vi "Periodic Tasks.vi"(8 "error in":errorcluster) -> ()   [LabVIEW 2019]
doc: "This VI runs in parallel to other tasks. It can contain as many user-defined periodic loops as you need. These can carry out PID or other sorts of timed response."
uses:
  <vilib>/Rock Robotics/WPI/Utilities/WPI_GetSetVariantRefNum.vi
  Robot Global Data.vi
  <vilib>/Rock Robotics/Network Tables/NT Read Boolean.vi
  <vilib>/Rock Robotics/WPI/RobotDrive/WPI_RobotDriveArcadeDrive_Standard(NoSaturation).vi
  <vilib>/Rock Robotics/Network Tables/NT Read Number.vi
  <vilib>/Rock Robotics/Network Tables/NT Write Numeric Array.vi
panel:
  in  "Target Y":dbl=1.0
  in  "Proportional Gain (X and Y)":dbl=0.25
  in  "Target X":dbl=1.0
  out "output":T1
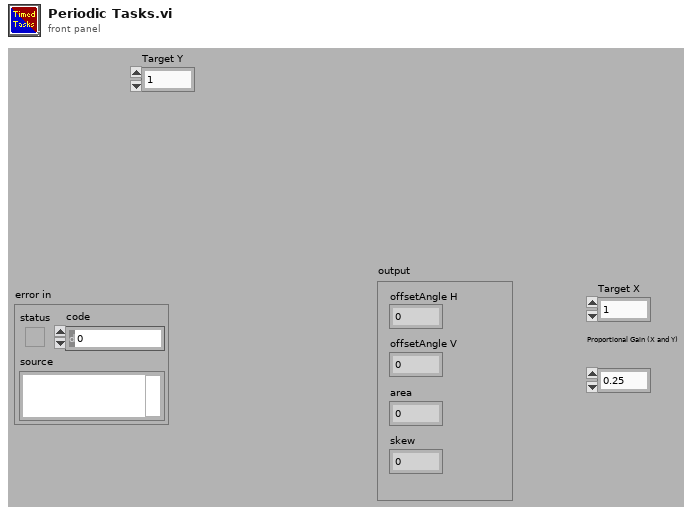
[diagram p1: front panel]
types:
  T1 = cluster{"offsetAngle H":dbl, "offsetAngle V":dbl, "area":dbl, "skew":dbl}
  T2 = typedef "WPI_JoystickDevRef.ctl" = cluster{"Device":T3}
  T3 = typedef "WPI_JoystickDeviceEnum.ctl" = enum16{"USB 0", "USB 1", "USB 2", "USB 3", "USB 4", "USB 5"}
  T4 = typedef "WPI_RobotDriveDevRef.ctl" = cluster{"DevStatus":errorcluster, "Motors[]":T5[], "Square Inputs":bool, "Max Output":dbl}
  T5 = typedef "WPI_MotorControlDeviceRef.ctl" = cluster{"DeviceStatus":errorcluster, "Type":T6, "PWM":cluster{"PWM Channel":T7, "DeadBand":T8}, "CAN":cluster{"Device Number":u8, "SetOutput VI Ref":variant, "GetOutput VI Ref":variant, "Enable VI Ref":variant, "Disable VI Ref":variant, "Data":variant}, "Invert":bool, "DIO PWM":cluster{"PWM \"Enable\" Channel":T7, "DIOChannel":T9, "PWM Rate":dbl}}
  T6 = typedef "WPI_MotorControlType.ctl" = enum16{"PWM", "CAN", "DIO PWM"}
  T7 = typedef "FPGA_DIOPWMChannel.ctl" = enum8{"PWM 0", "PWM 1", "PWM 2", "PWM 3", "PWM 4", "PWM 5", "PWM 6", "PWM 7", "PWM 8", "PWM 9", "PWM MXP 0", "PWM MXP 1", "PWM MXP 2", "PWM MXP 3", "PWM MXP 4", "PWM MXP 5", "PWM MXP 6", "PWM MXP 7", "PWM MXP 8", "PWM MXP 9", "Invalid"}
  T8 = typedef "WPI_PWMDeadband.ctl" = cluster{"Name":string, "maxPositivePwm":i32, "minPositivePwm":i32, "centerPwm":i32, "maxNegativePwm":i32, "minNegativePwm":i32, "angularRange":u16}
  T9 = typedef "FPGA_DIOChannel.ctl" = enum8{"DIO 0", "DIO 1", "DIO 2", "DIO 3", "DIO 4", "DIO 5", "DIO 6", "DIO 7", "DIO 8", "DIO 9", "DIO MXP 0", "DIO MXP 1", "DIO MXP 2", "DIO MXP 3", "DIO MXP 4", "DIO MXP 5", "DIO MXP 6", "DIO MXP 7", "DIO MXP 8", "DIO MXP 9", "DIO MXP 10", "DIO MXP 11", "DIO MXP 12", "DIO MXP 13", "DIO MXP 14", "DIO MXP 15", "SPI Port CS1", "SPI Port CS2", "SPI Port CS3", "SPI Port MISO", "SPI Port MOSI", "Invalid"}
  T10 = cluster{"JoystickDevRef":T2, "RobotDriveDevRef":T4}
  T11 = typedef "WPI_ServoDeviceRef.ctl" = cluster{"DeviceStatus":errorcluster, "PWM Channel":T7, "DeadBand":T8}
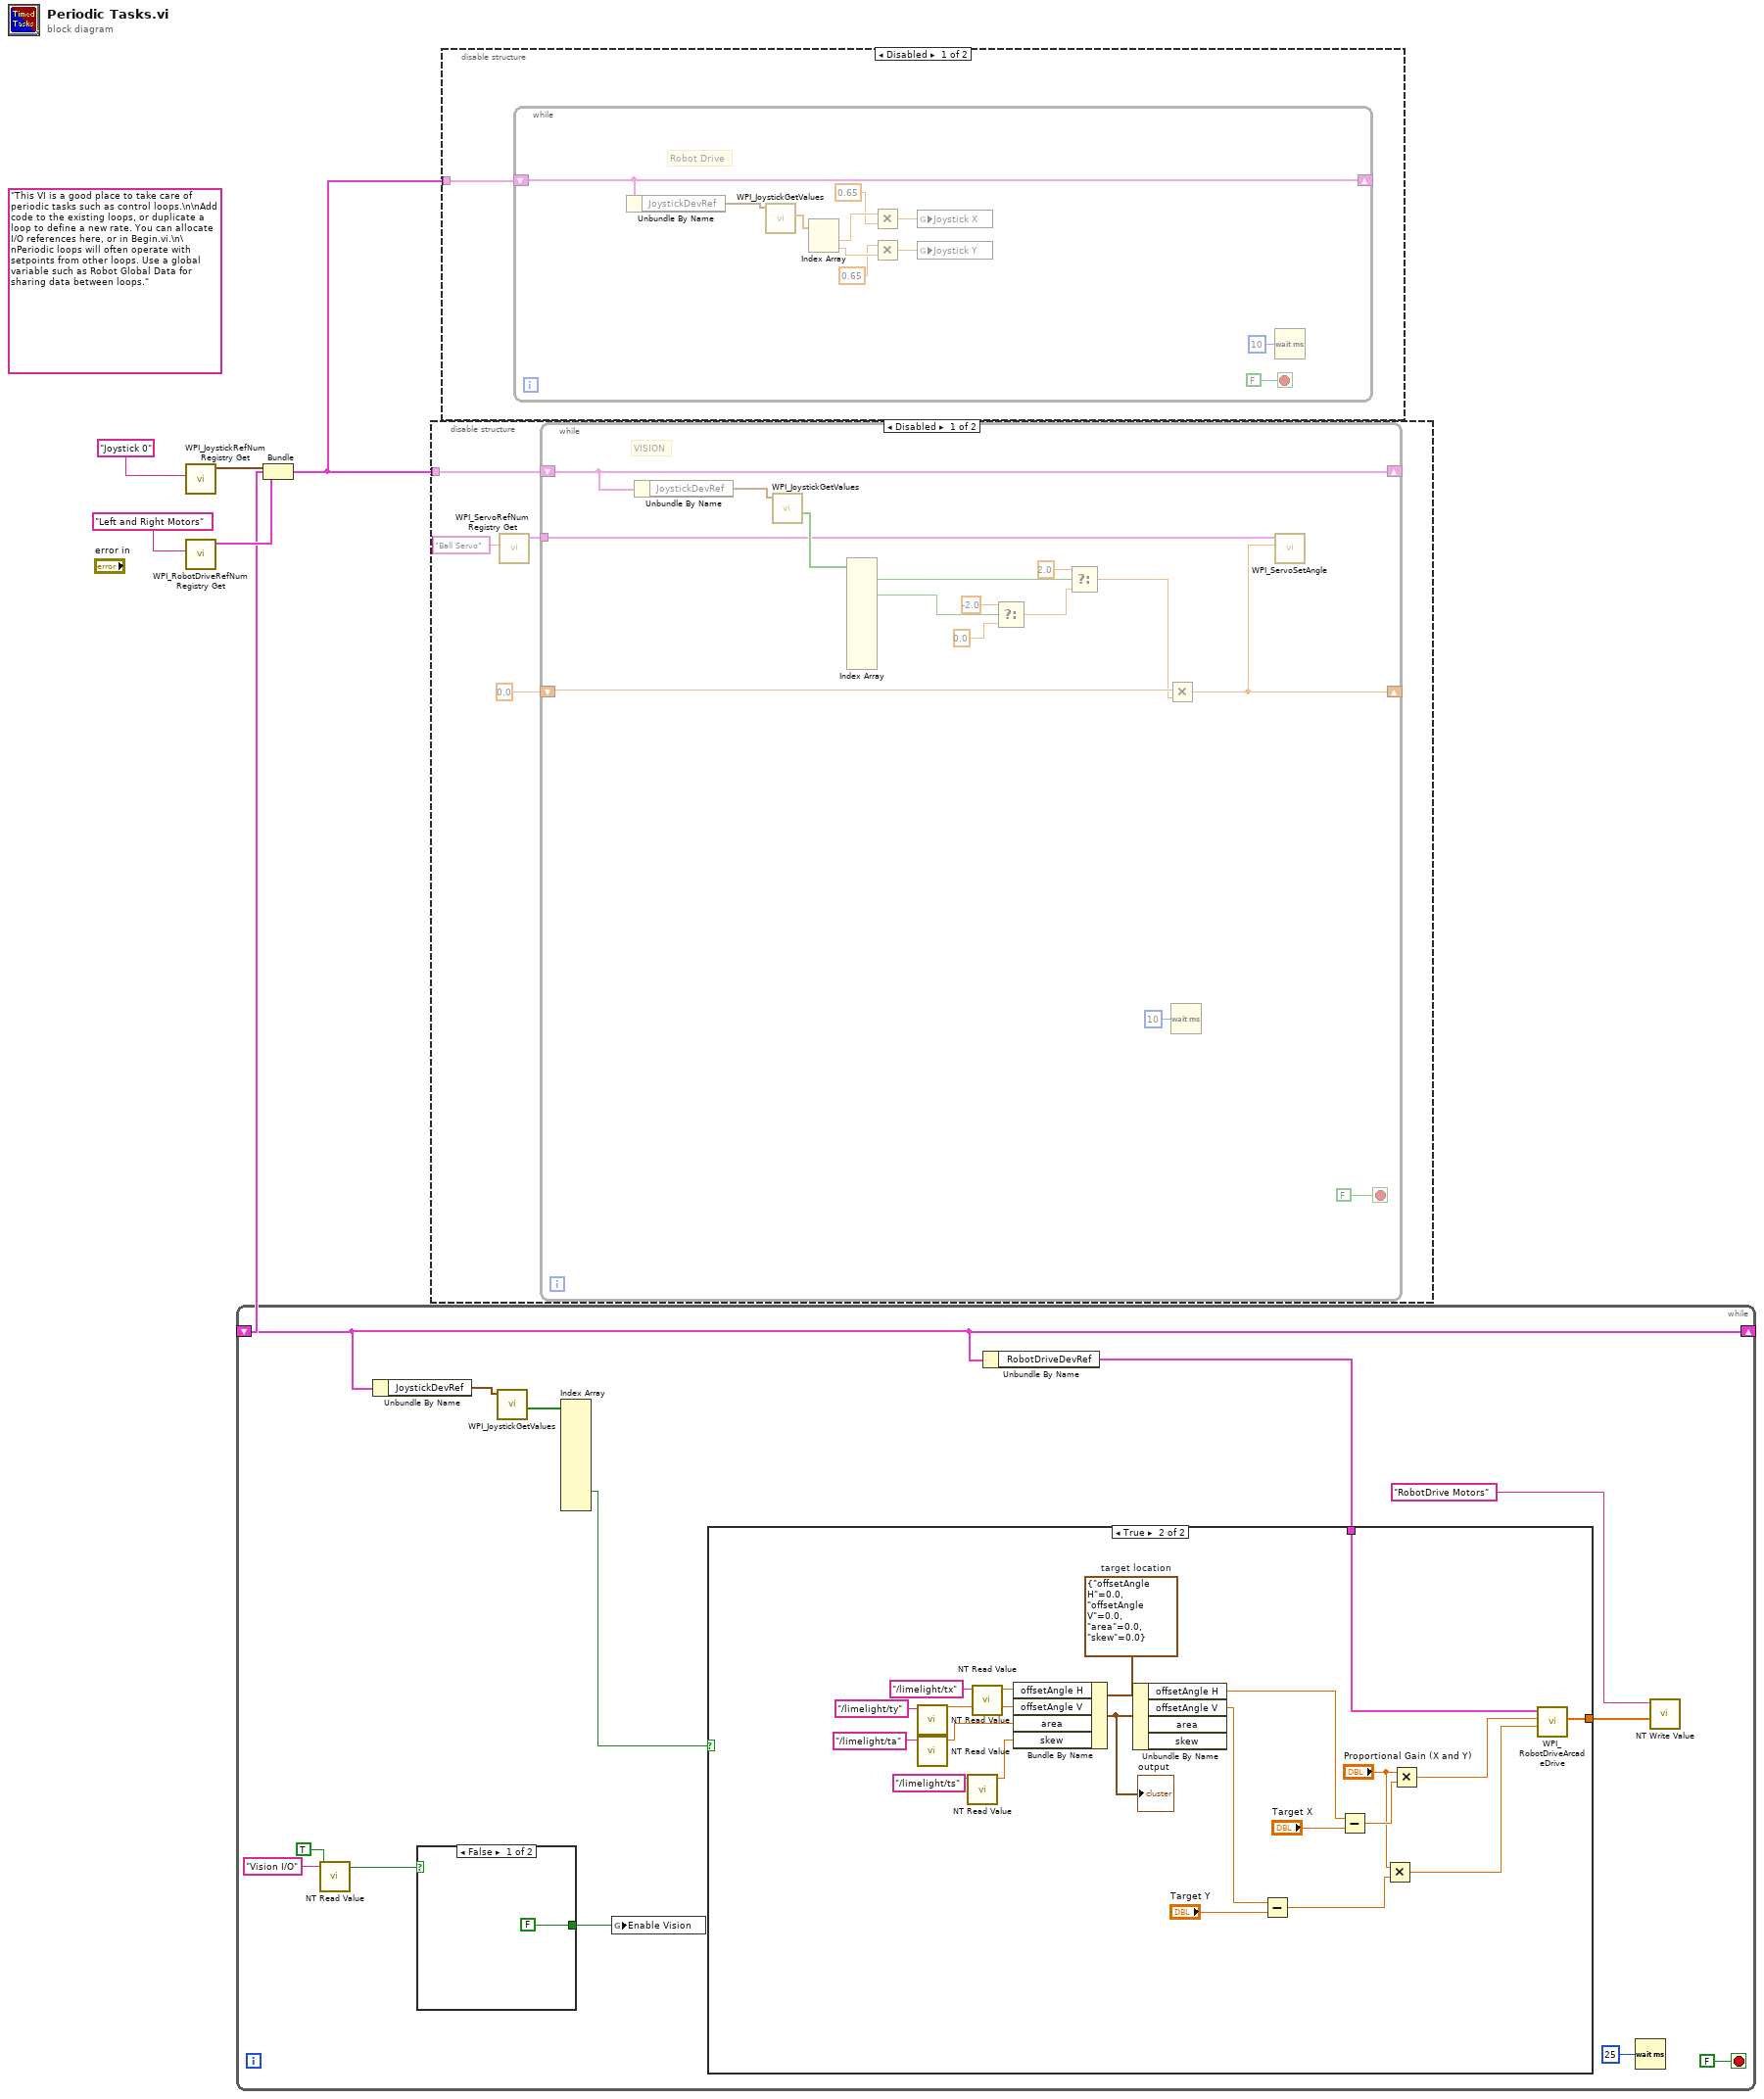
[diagram p0: block diagram]
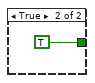
[diagram p4: hidden frame]
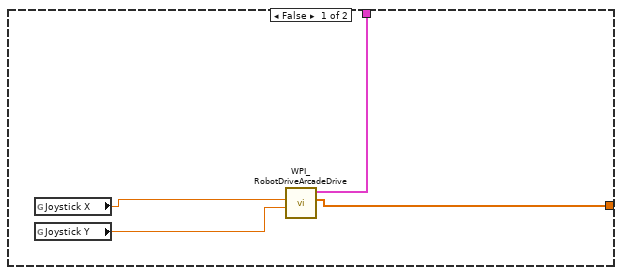
[diagram p5: hidden frame]
diagram:
  (unwired) "This VI is a good place to take care of periodic tasks such as control loops.\n\nAdd code to the existing loops, or duplicate a loop to define a new rate. You can allocate I/O references here, or in Begin.vi.\n\nPeriodic loops will often operate with setpoints from other loops. Use a global variable such as Robot Global Data for sharing data between loops."
  n1 = call <vilib>:"WPI_JoystickRefNum Registry Get.vi"("refnum name"="Joystick 0") -> ("JoystickDevRef"=w3:T2)  [unwired: 1 in, 9 out]
  n2 = call <vilib>:"WPI_RobotDriveRefNum Registry Get.vi"("refnum name"="Left and Right Motors") -> ("RobotDriveDevRef"=w2:T4)  [unwired: 1 in, 9 out]
  n3 = Bundle("JoystickDevRef"=w3, "RobotDriveDevRef"=w2) -> (w1:T10)  [unwired: 1 out]
  n4 = while {
    shift-right: [w16] -> _
    shift-left: w1 -> [w16]
    stop <- FALSE stop-if-true
    n5 = call-poly <vilib>:"NT Read Value.vi"("Default Value"=TRUE, "Name"="Vision I/O") -> ("Boolean"=w7:bool)  [unwired: 8 in, 1 out]
    n6 = Unbundle By Name(w16) -> ("JoystickDevRef"=w15:T2)
    n7 = case shown="False" w7 {
      tunnel: [FALSE ("Enable Vision") TRUE ("Enable Vision")] -> w6
      frame False {
      }
      frame True {
      }
    }
    n8 = call <vilib>:"WPI_JoystickGetValues.vi"("JoystickDevRef"=w15) -> ("Buttons"=w14:bool[])  [unwired: 6 in, 4 out]
    n9 = Index Array(array=w14) -> (element #10=w10:bool)  [unwired: 12 in, 11 out]
    n10 = global write "Robot Global Data.vi" "Enable Vision"(w6) -> ()
    n11 = Unbundle By Name(w16) -> ("RobotDriveDevRef"=w13:T4)
    n12 = case shown="True" w10 {
      tunnel: w13 -> [w24 w45]
      tunnel: [w21 w43] -> w11
      frame False {
        n13 = global read "Robot Global Data.vi" "Joystick X"() -> (w23:dbl)
        n14 = global read "Robot Global Data.vi" "Joystick Y"() -> (w22:dbl)
        n15 = call-poly <vilib>:"WPI_RobotDriveArcadeDrive.vi"("Y axis value"=w22, "X axis value"=w23, "RobotDriveDevRef"=w24) -> ("Motor Values"=w21:dbl[])  [unwired: 6 in, 2 out]
      }
      frame True {
        w36 = T1 {"offsetAngle H"=0.0, "offsetAngle V"=0.0, "area"=0.0, "skew"=0.0}  # target location
        n16 = call-poly <vilib>:"NT Read Value.vi"("Name"="/limelight/ty") -> ("Numeric"=w33:dbl)  [unwired: 9 in, 1 out]
        n17 = call-poly <vilib>:"NT Read Value.vi"("Name"="/limelight/ta") -> ("Numeric"=w32:dbl)  [unwired: 9 in, 1 out]
        n18 = call-poly <vilib>:"NT Read Value.vi"("Name"="/limelight/ts") -> ("Numeric"=w31:dbl)  [unwired: 9 in, 1 out]
        n19 = call-poly <vilib>:"NT Read Value.vi"("Name"="/limelight/tx") -> ("Numeric"=w41:dbl)  [unwired: 9 in, 1 out]
        n20 = Bundle By Name(cluster=w36, "offsetAngle H"=w41, "offsetAngle V"=w33, "area"=w32, "skew"=w31) -> (w42:T1)
        "output" <- w42
        n21 = Unbundle By Name(w42) -> ("offsetAngle H"=w35:dbl, "offsetAngle V"=w29:dbl)  [unwired: 2 out]
        n22 = Subtract(x=w29, y="Target Y") -> (x-y=w26:dbl)
        n23 = Subtract(x=w35, y="Target X") -> (x-y=w44:dbl)
        n24 = Multiply(x="Proportional Gain (X and Y)", y=w26) -> (x*y=w25:dbl)
        n25 = Multiply(x="Proportional Gain (X and Y)", y=w44) -> (x*y=w30:dbl)
        n26 = call-poly <vilib>:"WPI_RobotDriveArcadeDrive.vi"("Y axis value"=w25, "X axis value"=w30, "RobotDriveDevRef"=w45) -> ("Motor Values"=w43:dbl[])  [unwired: 6 in, 2 out]
      }
    }
    n27 = Wait (ms)(milliseconds to wait=u32 25) -> ()  [unwired: 1 out]
    n28 = call-poly <vilib>:"NT Write Value.vi"("Numeric Array"=w11, "Name"="RobotDrive Motors") -> ()  [unwired: 9 in, 1 out]
  }
  n29 = disable-structure shown="Disabled" {
    disable-tunnel: w1 -> [w49 _]
    frame Disabled {
      n30 = call <vilib>:"WPI_ServoRefNum Registry Get.vi"("refnum name"="Ball Servo") -> ("ServoDeviceRef"=w48:T11)  [unwired: 9 in, 1 out]
      n31 = while {
        shift-right: [w63] -> _
        shift-left: w49 -> [w63]
        tunnel: w48 -> [w59]
        shift-right: [w50] -> _
        shift-left: 0.0 -> [w58]
        stop <- FALSE stop-if-true
        # "VISION"
        n32 = Unbundle By Name(w63) -> ("JoystickDevRef"=w62:T2)
        n33 = call <vilib>:"WPI_JoystickGetValues.vi"("JoystickDevRef"=w62) -> ("Buttons"=w61:bool[])  [unwired: 6 in, 4 out]
        n34 = Index Array(array=w61) -> (element #1=w57:bool, element #3=w56:bool)  [unwired: 12 in, 10 out]
        n35 = Select(t=-2.0, s=w56, f=0.0) -> (s? t:f=w52:dbl)
        n36 = Select(t=2.0, s=w57, f=w52) -> (s? t:f=w51:dbl)
        n37 = Multiply(x=w58, y=w51) -> (x*y=w50:dbl)
        n38 = Wait (ms)(milliseconds to wait=u32 10) -> ()  [unwired: 1 out]
        n39 = call <vilib>:"WPI_ServoSetAngle.vi"("Angle"=w50, "ServoDeviceRef"=w59) -> ()  [unwired: 8 in, 2 out]
      }
    }
    frame Enabled {
    }
  }
  n40 = disable-structure shown="Disabled" {
    disable-tunnel: w1 -> [w65 _]
    frame Disabled {
      n41 = while {
        shift-right: [w75] -> _
        shift-left: w65 -> [w75]
        stop <- FALSE stop-if-true
        # "Robot Drive"
        n42 = Unbundle By Name(w75) -> ("JoystickDevRef"=w73:T2)
        n43 = call <vilib>:"WPI_JoystickGetValues.vi"("JoystickDevRef"=w73) -> ("Axes"=w72:dbl[])  [unwired: 6 in, 4 out]
        n44 = Index Array(array=w72) -> (element #1=w71:dbl, element #2=w69:dbl)  [unwired: 2 in]
        n45 = Multiply(x=w71, y=0.65) -> (x*y=w67:dbl)
        n46 = Multiply(x=0.65, y=w69) -> (x*y=w66:dbl)
        n47 = global write "Robot Global Data.vi" "Joystick X"(w67) -> ()
        n48 = global write "Robot Global Data.vi" "Joystick Y"(w66) -> ()
        n49 = Wait (ms)(milliseconds to wait=u32 10) -> ()  [unwired: 1 out]
      }
    }
    frame Enabled {
    }
  }
